vi "Select Controller Objects.vi"(10 "Outputs":T1, 11 "Inputs":T2) -> (2 "Session":refnum<class "Session.lvclass">, 3 "Response":refnum<class "Response.lvclass">, 5 "Response?":bool, 7 "Trace Message":string)   [LabVIEW 2020, in "HTTP Server.lvlib" / "Server.lvclass"]
uses:
  Server.lvclass
  Controller Inputs.ctl
  Values/Values.lvclass
  <vilib>/IlluminatedG/IG HTTP Utils/HTTP Utils/Request/Request.lvclass
  Session/Session.lvclass
  Controller Outputs.ctl
  <vilib>/IlluminatedG/IG HTTP Utils/HTTP Utils/Response/Response.lvclass
  Server.lvclass/Server.ctl
  HTTP Server.lvlib
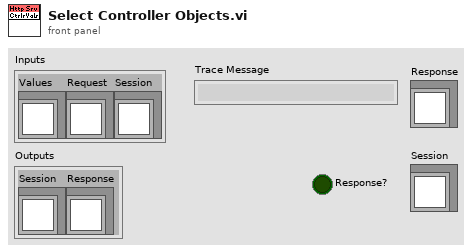
[diagram p1: front panel]
types:
  T1 = typedef "HTTP Server.lvlib/Controller Outputs.ctl" = cluster{"Session":refnum<class "Session.lvclass">, "Response":refnum<class "Response.lvclass">}
  T2 = typedef "HTTP Server.lvlib/Controller Inputs.ctl" = cluster{"Values":refnum<class "Values.lvclass">, "Request":refnum<class "Request.lvclass">, "Session":refnum<class "Session.lvclass">}
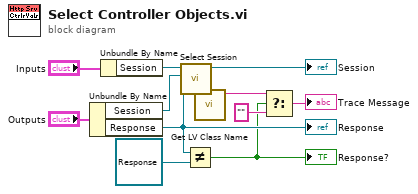
[diagram p0: block diagram]
diagram:
  n1 = Unbundle By Name("Outputs") -> ("Session"=w8:refnum<class "Session.lvclass">, "Response"=w5:refnum<class "Response.lvclass">)
  "Response" <- w5
  n2 = Unbundle By Name("Inputs") -> ("Session"=w9:refnum<class "Session.lvclass">)
  n3 = call "Select Session.vi"("Output Session"=w8, "Input Session"=w9) -> ("Session"=→"Session":refnum<class "Session.lvclass">)  [unwired: 9 in]
  n4 = Not Equal?(x=w5, y=refnum<class "Response.lvclass"> refnum) -> (x != y?=w2:bool)
  "Response?" <- w2
  n5 = call <vilib>:"Get LV Class Name.vi"("object"=w5) -> ("class name"=w4:string)  [unwired: 9 in, 1 out]
  n6 = Select(t=w4, s=w2, f="") -> (s? t:f=→"Trace Message":string)
